vi "Deduplication2DArray.vi"(11 "array":string[][](array[string])) -> (3 "result":string[][](array[string]))   [LabVIEW 2018, in "Library-Ctrl.lvlib"]
uses:
  Library-Ctrl.lvlib
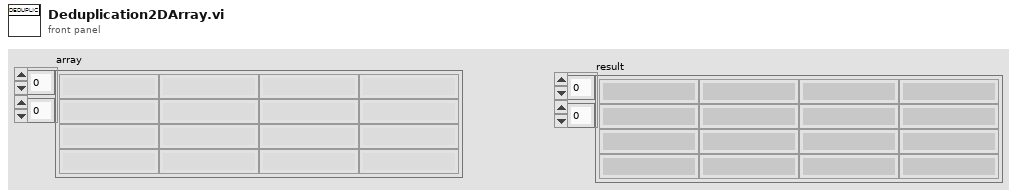
[diagram p1: front panel]
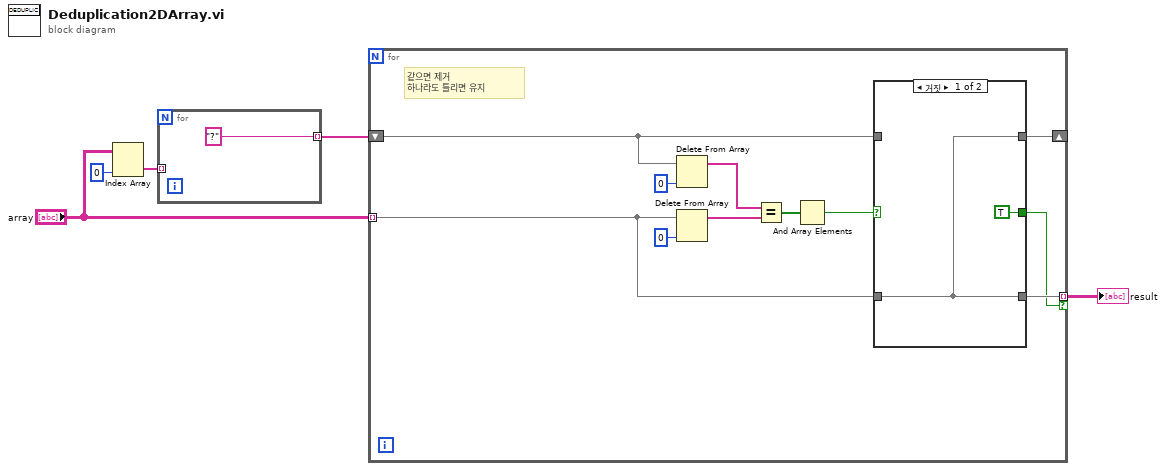
[diagram p0: block diagram]
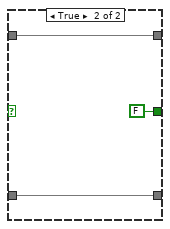
[diagram p2: hidden frame]
diagram:
  n1 = Index Array(array="array", index (col)=0 ("비활성화된 인덱스 (열)")) -> (element=w2:string[])  [unwired: 1 in]
  n2 = for {
    tunnel: w2 -> [_] mode=indexing
    tunnel: ["?"] -> w1 mode=indexing
  }
  n3 = for {
    tunnel: "array" -> [w13] mode=indexing
    shift-right: [w10] -> _
    shift-left: w1 -> [w14]
    tunnel: [w12] -> w5 mode=indexing if=w11
    # "같으면 제거\n하나라도 틀리면 유지"
    n4 = Delete From Array(array=w14, index=0 ("인덱스")) -> (array with subset deleted=w8:string[])  [unwired: 1 in, 1 out]
    n5 = Delete From Array(array=w13, index=0 ("인덱스")) -> (array with subset deleted=w15:string[])  [unwired: 1 in, 1 out]
    n6 = Equal?(x=w8, y=w15) -> (x = y?=w9:bool[])
    n7 = And Array Elements(Boolean array=w9) -> (logical AND=w7:bool)
    n8 = case shown="거짓" w7 {
      tunnel: w14 -> [_ w21]
      tunnel: w13 -> [w19 w22]
      tunnel: [w19 w22] -> w12
      tunnel: [TRUE FALSE] -> w11
      tunnel: [w19 w21] -> w10
      frame False {
      }
      frame True {
      }
    }
  }
  "result" <- w5
